vi "Joystick Error Filter.vi"(1 "Axis":dbl) -> (0 "Filtered Axis":dbl)   [LabVIEW 2013]
panel:
  # "Filters Out Extremly Small Values"
  # "that occur sometimes instead of 0 on the logitech extreme 3D joystick"
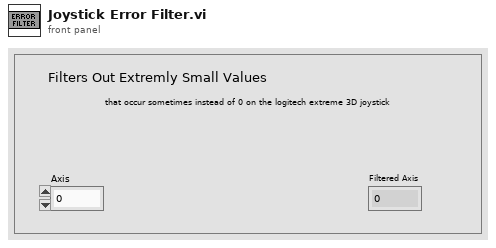
[diagram p1: front panel]
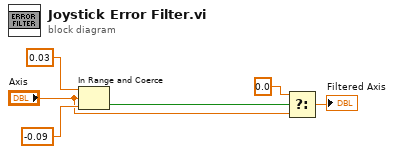
[diagram p0: block diagram]
diagram:
  n1 = In Range and Coerce(upper limit=0.03, x="Axis", lower limit=-0.09 ("upper limit")) -> (In Range?=w3:bool)  [unwired: 1 out]
  n2 = Select(t=0.0, s=w3, f="Axis") -> (s? t:f=→"Filtered Axis":dbl)
